vi "StateMachine.vi"() -> ()   [LabVIEW 2014]
uses:
  Controls/StateControl.ctl
  <vilib>/MakerHub/LINX/LMH-LINX.lvlib
  <vilib>/MakerHub/LINX/Public/Peripherals/PWM/PWM Set Duty Cycle 1 Chan.vi
  <vilib>/MakerHub/LINX/Public/Peripherals/Digital/Digital Write 1 Chan.vi
  <vilib>/MakerHub/LINX/Public/Utilities/Open Local.vi
panel:
  out "find list":string[](array[string])
  in  "DO Channel":u8=7
  in  "stop":bool
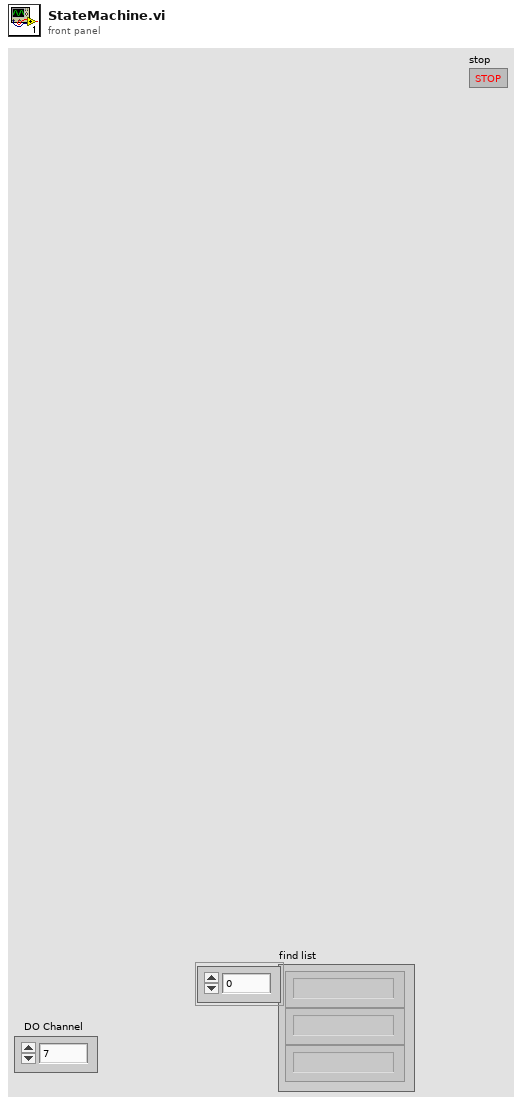
[diagram p1: front panel]
types:
  T1 = typedef "StateControl.ctl" = enum16{"IDLE", "PROCESS SCAN", "RESET"}
  T2 = typedef "LMH-LINX.lvlib/LINX Ref.ctl" = cluster{"IO":T3, "Interface":T4, "LINX Device Config":T5}
  T3 = typedef "LMH-LINX.lvlib/Platform.ctl" = enum16{"Remote", "Local"}
  T4 = typedef "LMH-LINX.lvlib/Interface.ctl" = enum16{"Serial", "TCP"}
  T5 = typedef "LMH-LINX.lvlib/Device.lvlib/LINX Device Config.ctl" = cluster{"Interface":T4, "COM Port":refnum<visa-resource-name>, "TCP Configuration":T6, "Device Family":u8, "Device ID":u8, "Device Name":string, "TCP Ref":refnum<k5>, "Channels":T7}
  T6 = typedef "LMH-LINX.lvlib/Device.lvlib/TCP Config.ctl" = cluster{"IP Address":string, "Port":u16}
  T7 = typedef "LMH-LINX.lvlib/Channels.ctl" = cluster{"DI":u8[], "DO":u8[], "AI":u8[], "AO":u8[], "PWM":u8[], "QE":u8[], "UART":u8[], "I2C 2":u8[], "SPI":u8[], "CAN":u8[], "Servo":u8[], "AI Ref (V)":dbl, "AI Resolution (Bits)":u8, "AO Ref (V)":dbl, "AO Resolution (Bits)":u8}
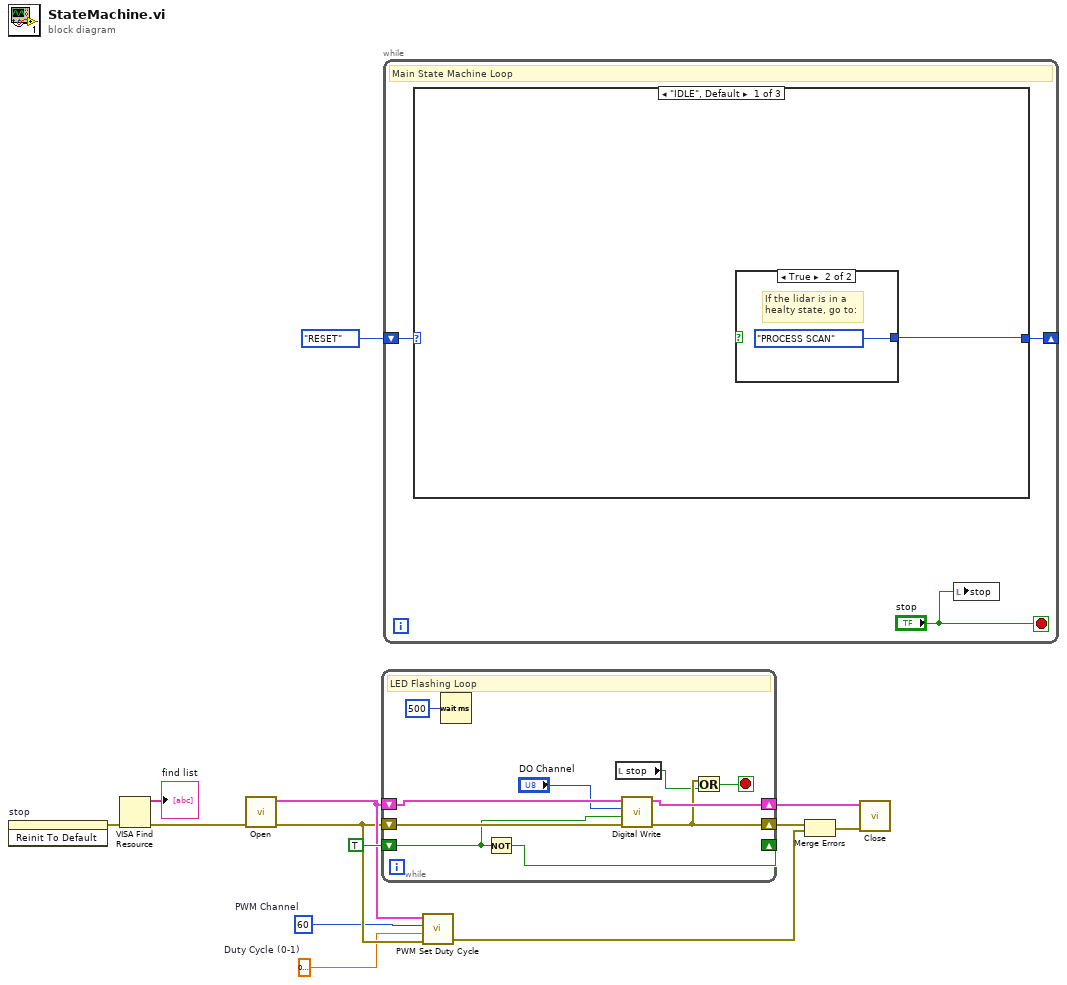
[diagram p0: block diagram]
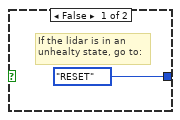
[diagram p2: hidden frame]
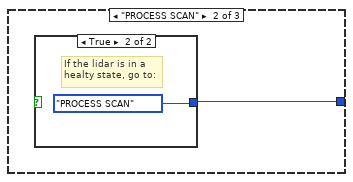
[diagram p3: hidden frame]
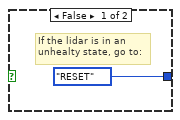
[diagram p4: hidden frame]
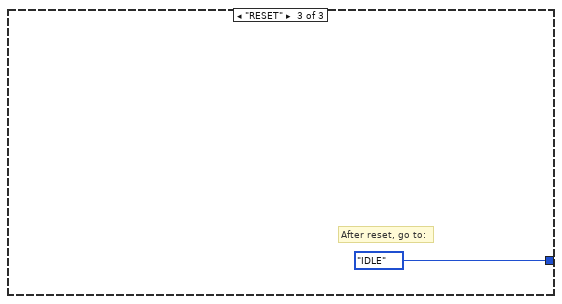
[diagram p5: hidden frame]
diagram:
  w2 = 0.9999999999999999  # Duty Cycle (0-1)
  w3 = u8 60  # PWM Channel
  n1 = invoke on="stop" class="Bool" method="Reinit To Default"() -> (error out=w1:errorcluster)  [unwired: 3 in, 2 out]
  n2 = VISA Find Resource(8:w1) -> (0:w11:errorcluster, 3:→"find list":string[])  [unwired: 2 in, 1 out]
  n3 = call-poly <vilib>:"Open.vi"("Error In"=w11) -> ("Error Out"=w4:errorcluster, "LINX Resource"=w5:T2)  [unwired: 8 in, 1 out]
  n4 = while {
    shift-right: [w22] -> w9
    shift-left: w5 -> [w23]
    shift-right: [w20] -> w8
    shift-left: w4 -> [w21]
    shift-right: [w17] -> _
    shift-left: TRUE -> [w16]
    stop <- w15 stop-if-true
    # "LED Flashing Loop"
    n5 = Wait (ms)(milliseconds to wait=u32 500) -> ()  [unwired: 1 out]
    n6 = Not(x=w16) -> (.not. x?=w17:bool)
    n7 = local read "stop"() -> (w14:bool)
    n8 = call-poly <vilib>:"Digital Write.vi"("Error In"=w21, "Output Value"=w16, "DO Channel"="DO Channel", "LINX Resource"=w23) -> ("Error Out"=w20:errorcluster, "LINX Resource"=w22:T2)  [unwired: 6 in]
    n9 = Or(x=w20, y=w14) -> (x .or. y?=w15:bool)
  }
  n10 = while {
    shift-right: [w25] -> _
    shift-left: StateControl."RESET" -> [w26]
    stop <- "stop" stop-if-true
    # "Main State Machine Loop"
    n11 = case shown="\"IDLE\", Default" w26 {
      tunnel: [w27 w30 StateControl."IDLE"] -> w25
      frame "IDLE", Default {
        n12 = case shown="True" {
          selector: _ -> [_ _]
          tunnel: [StateControl."RESET" StateControl."PROCESS SCAN"] -> w27
          frame False {
            # "If the lidar is in an \nunhealty state, go to:"
          }
          frame True {
            # "If the lidar is in a \nhealty state, go to:"
          }
        }
      }
      frame "PROCESS SCAN" {
        n13 = case shown="True" {
          selector: _ -> [_ _]
          tunnel: [StateControl."RESET" StateControl."PROCESS SCAN"] -> w30
          frame False {
            # "If the lidar is in an \nunhealty state, go to:"
          }
          frame True {
            # "If the lidar is in a \nhealty state, go to:"
          }
        }
      }
      frame "RESET" {
        # "After reset, go to:"
      }
    }
    n14 = local write "stop"("stop") -> ()
  }
  n15 = call-poly <vilib>:"PWM Set Duty Cycle.vi"("Error In"=w4, "Duty Cycle (0-1)"=w2, "PWM Channel"=w3, "LINX Resource"=w5) -> ("Error Out"=w6:errorcluster)  [unwired: 6 in, 1 out]
  n16 = Merge Errors(w8, w6) -> (w7:errorcluster)
  n17 = call <vilib>:"Close.vi"("Error In"=w7, "LINX Resource"=w9) -> ()  [unwired: 9 in, 1 out]
